vi "Configure and Start Acoustic AI.vi"(8 "error in":errorcluster, 11 "cPAS in":refnum<class "cPAS.lvclass">) -> (0 "error out":errorcluster, 3 "cPAS out":refnum<class "cPAS.lvclass">)   [LabVIEW 2015, in "cPAS.lvclass"]
doc: "Configure and start the high frequency task for collecting the data microphone and/or photodiode data. The default VI starts a task named PAS Laser AI and stuffs it into the variable <b>acoustic</b>."
uses:
  cPAS.lvclass
  Reusable/PAS/Main/Controls/LasLam.ctl
  Reusable/PAS/Main/Controls/Cell Condition.ctl
  cPAS.lvclass/cPAS.ctl
  Reusable/PAS/Main/Read Cells.vi
  Reusable/PAS/Cell/Write extParams.vi
  Reusable/PAS/Cell/Write l (nm).vi
  Reusable/PAS/Cell/Write Condition.vi
  Reusable/PAS/Main/Write Cells.vi
  Reusable/PAS/Cell/PAS Cell.lvclass
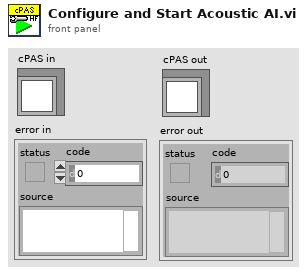
[diagram p1: front panel]
types:
  T1 = typedef "Cell Condition.ctl" = enum16{"Dry", "Humidified", "Denuded"}
  T2 = typedef "LasLam.ctl" = enum16{"405", "532", "661"}
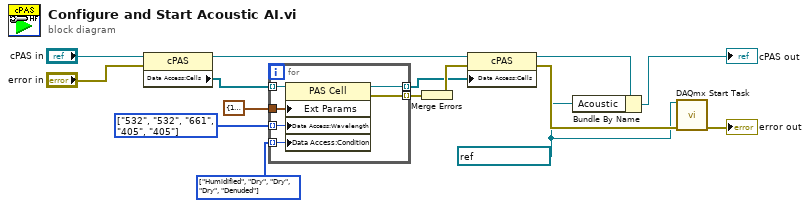
[diagram p0: block diagram]
diagram:
  w1 = refnum<k21> "PAS Laser AI" ("Acoustic")
  w4 = T1[] [enum."Humidified", enum."Dry", enum."Dry", enum."Dry", enum."Denuded"] items=["Dry", "Humidified", "Denuded"]
  w5 = T2[] [enum."532", enum."532", enum."661", enum."405", enum."405"] items=["405", "532", "661"]
  n1 = property class="cPAS"(reference="cPAS in", error in="error in") -> (reference out=w10:refnum<class "cPAS.lvclass">, "Data Access:Cells"=w7:refnum<class "PAS Cell.lvclass">[])  [unwired: 1 out]
  n2 = for {
    tunnel: [w21] -> w9 mode=indexing
    tunnel: w7 -> [w20] mode=indexing
    tunnel: cluster{"slope":sgl, "zero":sgl} {"slope"=1.0, "zero"=0.0} ("Ext Params") -> [w19]
    tunnel: w5 -> [w18] mode=indexing
    tunnel: w4 -> [w17] mode=indexing
    tunnel: [w16] -> w3 mode=indexing
    n3 = property class="PAS Cell"(reference=w20, "Ext Params"=w19, "Data Access:Wavelength"=w18, "Data Access:Condition"=w17) -> (reference out=w16:refnum<class "PAS Cell.lvclass">, error out=w21:errorcluster)  [unwired: 1 in]
  }
  n4 = Merge Errors(w9) -> (w8:errorcluster)
  n5 = property class="cPAS"(reference=w10, error in=w8, "Data Access:Cells"=w3) -> (reference out=w13:refnum<class "cPAS.lvclass">, error out=w12:errorcluster)
  n6 = Bundle By Name(cluster=w13, "Acoustic"=w1) -> (→"cPAS out":refnum<class "cPAS.lvclass">)
  n7 = call <vilib>:"DAQmx Start Task.vi"("task/channels in"=w1, "error in"=w12) -> ("error out"=→"error out":errorcluster)  [unwired: 12 in, 1 out]
